vi "Get Images Ref.vi"(8 "error in (no error)":errorcluster caption="错误输入（无错误）", 11 "ImageListClass 输入":refnum<class "ImageListClass.lvclass"> caption="DNL_LabVIEW Object in") -> (0 "error out":errorcluster caption="错误输出", 2 "Images":refnum<k24>, 3 "ImageListClass 输出":refnum<class "ImageListClass.lvclass"> caption="DNL_LabVIEW Object out")   [LabVIEW 2013, in "ImageListClass.lvclass"]
uses:
  ImageListClass.lvclass
  System.Windows.Forms
  ImageListClass.lvclass/ImageListClass.ctl
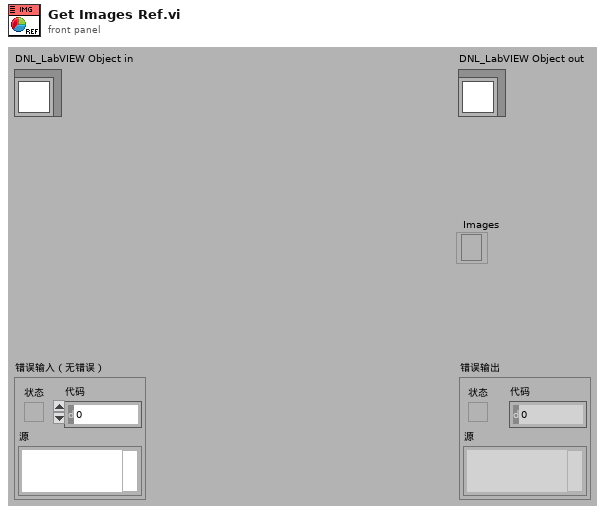
[diagram p1: front panel]
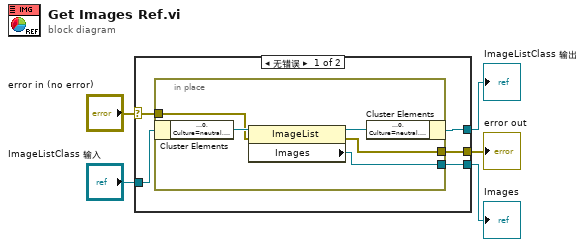
[diagram p0: block diagram]
diagram:
  n1 = case shown="无错误" "error in (no error)" {
    selector: "error in (no error)" -> [w7 w17]
    tunnel: [w6 w17] -> w4
    tunnel: [w8 w16] -> w2
    tunnel: "ImageListClass 输入" -> [w10 w16]
    tunnel: [w9 _] -> w1
    frame No Error {
      n2 = in-place {
        in-place-border: [w14] -> w9
        in-place-border: w7 -> [w12]
        in-place-border: [w11] -> w6
        n3 = in-place-cluster #1(w10) -> ("ImageList"=w15:refnum<k24>)
        n4 = property class="ImageList"(reference=w15, error in=w12) -> (reference out=w13:refnum<k24>, error out=w11:errorcluster, "Images"=w14:refnum<k24>)
        n5 = in-place-cluster #1("ImageList"=w13) -> (w8:refnum<class "ImageListClass.lvclass">)
      }
    }
    frame Error {
    }
  }
  "error out" <- w4
  "ImageListClass 输出" <- w2
  "Images" <- w1
